vi "timerforONR.vi"(5 "Boolean":bool) -> (6 "Numeric":dbl, 10 "Numeric 2":dbl)   [LabVIEW 2017]
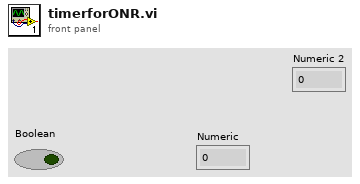
[diagram p1: front panel]
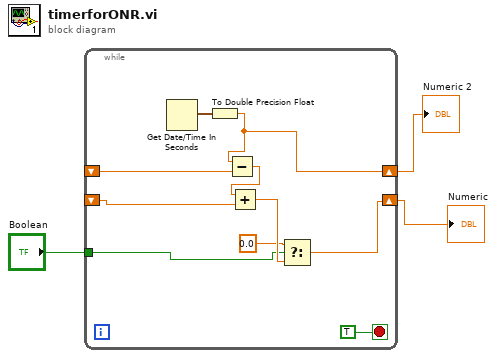
[diagram p0: block diagram]
diagram:
  n1 = while {
    shift-right: [w11] -> w1
    shift-left: _ -> [w12]
    shift-right: [w6] -> w2
    shift-left: _ -> [w9]
    tunnel: "Boolean" -> [w7]
    stop <- TRUE stop-if-true
    n2 = Get Date/Time In Seconds() -> (seconds since 1Jan1904=w13:timestamp)
    n3 = To Double Precision Float(number=w13) -> (double precision float=w11:dbl)
    n4 = Subtract(x=w11, y=w12) -> (x-y=w10:dbl)
    n5 = Add(x=w10, y=w9) -> (x+y=w8:dbl)
    n6 = Select(t=0.0, s=w7, f=w8) -> (s? t:f=w6:dbl)
  }
  "Numeric" <- w2
  "Numeric 2" <- w1
